vi "worksheet split panes.vi"(8 "error in (no error)":errorcluster, 9 "horizontal":dbl, 10 "vertical":dbl, 11 "worksheet":u32) -> (0 "error out":errorcluster, 3 "function return":u32(ring))   [LabVIEW 2015, in "xlsxwriter.lvlib"]
doc: "lxw_error worksheet_split_panes(lxw_worksheet worksheet, double vertical, double horizontal);"
uses:
  xlsxwriter.lvlib
  xlsxwriter.dll
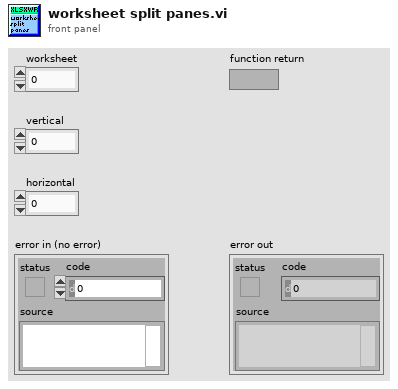
[diagram p1: front panel]
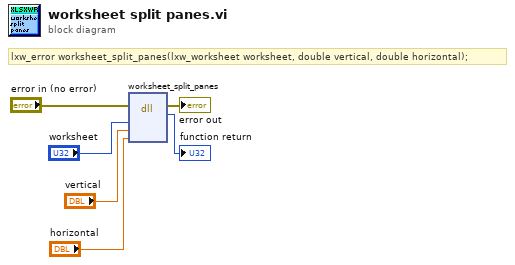
[diagram p0: block diagram]
diagram:
  # "lxw_error worksheet_split_panes(lxw_worksheet worksheet, double vertical, double horizontal);"
  n1 = dll-call lib="C:/Users/WDAGUtilityAccount/Desktop/lv_vis_added_cell/xlsxwriter.*" fn="worksheet_split_panes"(error in="error in (no error)", "worksheet"="worksheet", "vertical"="vertical", "horizontal"="horizontal") -> (error out=→"error out":errorcluster, →"function return":u32)  [unwired: 5 in, 1 out]
